vi "simulate arduino sensirion read to stream and log (sub-vi).vi"(0 "logfile refnum":refnum<file>, 1 "VISA resource name (COM3)":refnum<visa-resource-name>="COM3", 2 "stop channel":T1, 3 "abort? (F)":bool, 5 "read byte count (512)":u32=512, 7 "expected num sensors (12)":i32=12, 9 "baud rate (576000)":u32=576000, 11 "error in (no error)":errorcluster, 12 "dirty data? (F)":bool) -> (4 "logfile refnum out":refnum<file>, 8 "sensor data cluster channel":T2, 15 "error out":errorcluster)   [LabVIEW 2021]
uses:
  <extravilib>/ChannelInstances/Stream-t'sensirion_data_with_time.ctl'/)Channel.ctl
  type-defs/sensirion_data_with_time.ctl
  controls/sensirion_flow_sensor_data.ctl
  <extravilib>/ChannelInstances/Tag-bool/))Channel.ctl
  <extravilib>/ChannelInstances/Stream-t'sensirion_data_with_time.ctl'/Read With Abort.vi
  <extravilib>/ChannelInstances/Stream-t'sensirion_data_with_time.ctl'/Write With Abort.vi
  <extravilib>/ChannelInstances/Tag-bool/Read With Abort.vi
  <extravilib>/ChannelInstances/Tag-bool/Write With Abort.vi
  <extravilib>/ChannelInstances/Stream-t'sensirion_data_with_time.ctl'/EndpointRead.vi
  <extravilib>/ChannelInstances/Stream-t'sensirion_data_with_time.ctl'/Endpoint.vi
  <extravilib>/ChannelInstances/Tag-bool/EndpointRead.vi
  <extravilib>/ChannelInstances/Tag-bool/Endpoint.vi
  <extravilib>/ChannelInstances/Tag-bool/Instantiate.vi
  <extravilib>/ChannelInstances/Stream-t'sensirion_data_with_time.ctl'/Instantiate.vi
  <extravilib>/ChannelInstances/Stream-t'sensirion_data_with_time.ctl'/)Channel.vi
  <resource>/ChannelSupport/_ChannelSupport/WaitIfNeeded.vi
  <extravilib>/ChannelInstances/Stream-t'sensirion_data_with_time.ctl'.lvlib
  <extravilib>/ChannelInstances/Tag-bool.lvlib
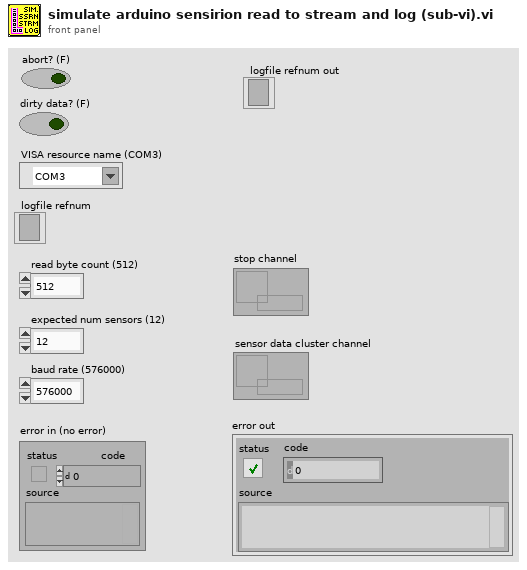
[diagram p1: front panel]
types:
  T1 = typedef "Tag-bool.lvlib/))Channel.ctl" = refnum<queue>
  T2 = typedef "Stream-t'sensirion_data_with_time.ctl'.lvlib/)Channel.ctl" = refnum<queue>
  T3 = typedef "sensirion_data_with_time.ctl" = cluster{"sensor data array":T4[], "relative timestamp":dbl, "error":errorcluster}
  T4 = typedef "sensirion_flow_sensor_data.ctl" = cluster{"flow rate \n":dbl[unit], "flow val. status":bool, "temperature":dbl[unit], "temp. val status":bool, "air in line?":bool, "high flow?":bool, "flag. val status":bool}
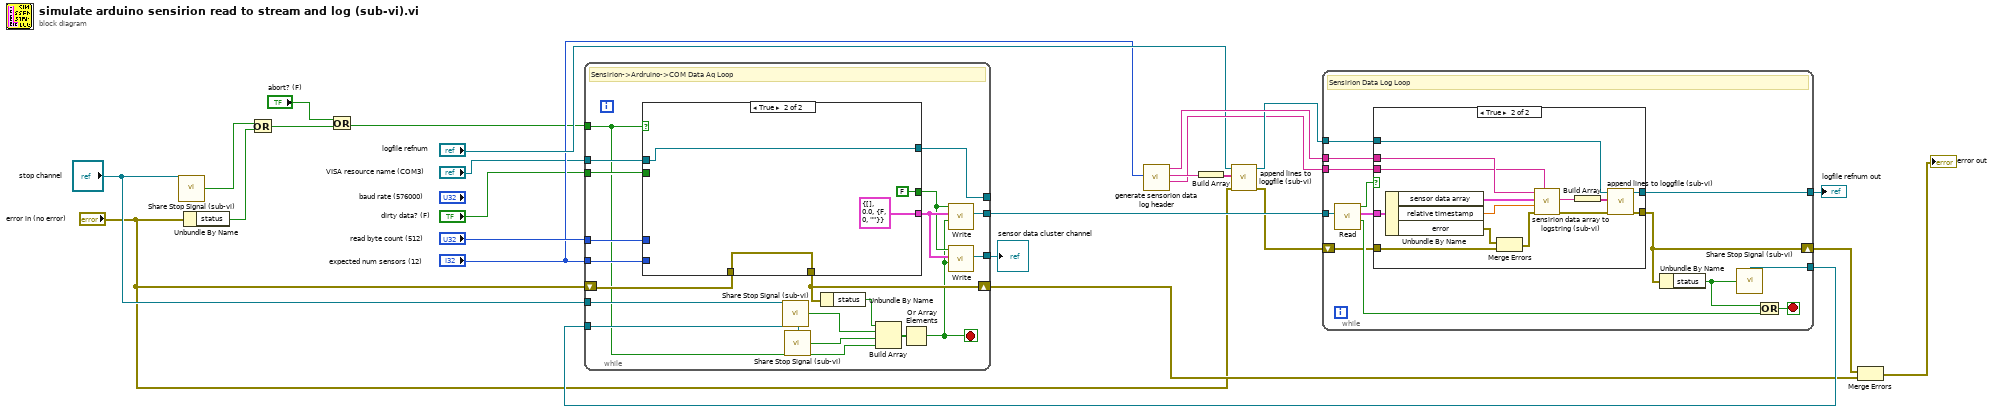
[diagram p0: block diagram]
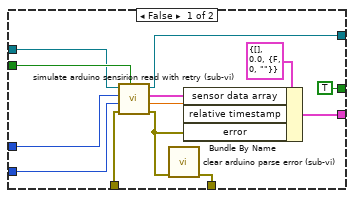
[diagram p3: hidden frame]
diagram:
  n1 = call "Share Stop Signal (sub-vi).vi"("channel"="stop channel") -> ("stop"=w8:bool)  [unwired: 1 in]
  n2 = Unbundle By Name("error in (no error)") -> ("status"=w9:bool)
  n3 = Or(x=w8, y=w9) -> (x .or. y?=w7:bool)
  n4 = Or(x="abort? (F)", y=w7) -> (x .or. y?=w4:bool)
  n5 = call "generate sensorion data log header.vi"("num sensors"="expected num sensors (12)") -> ("delimiter"=w16:string, "sensor data header string"=w25:string, "value format"=w22:string)  [unwired: 8 in]
  n6 = Build Array(w25) -> (w24:string[])
  n7 = call "append lines to loggfile (sub-vi).vi"("error in (no error)"="error in (no error)", "string array"=w24, "file refnum"="logfile refnum") -> ("error out"=w19:errorcluster, "file refnum out"=w21:refnum<file>)  [unwired: 7 in]
  n8 = while {
    tunnel: "read byte count (512)" -> [w44]
    tunnel: [w41] -> w23
    tunnel: "expected num sensors (12)" -> [w40]
    shift-right: [w37] -> w5
    shift-left: "error in (no error)" -> [w43]
    tunnel: [w39] -> w20
    tunnel: "stop channel" -> [w38]
    tunnel: [w36] -> _
    tunnel: w15 -> [w35]
    tunnel: "dirty data? (F)" -> [w34]
    tunnel: w4 -> [w28]
    tunnel: "VISA resource name (COM3)" -> [w33]
    stop <- w26 stop-if-true
    # "Sensirion->Ardruino->COM Data Aq Loop"
    n9 = case shown="True" w28 {
      tunnel: w44 -> [w57 _]
      tunnel: w43 -> [w47 w58]
      tunnel: [w53 T3 {"sensor data array"=[], "relative timestamp"=0.0, "error"={"status"=FALSE, "code"=0, "source"=""}} ("Cluster")] -> w42
      tunnel: w40 -> [w52 _]
      tunnel: [w45 w58] -> w37
      tunnel: [w51 w61] -> w36
      tunnel: w34 -> [w50 _]
      tunnel: w33 -> [w49 w61]
      tunnel: [TRUE ("element valid? (T)") FALSE ("element valid? (T)")] -> w32
      frame False {
        n10 = call "simulate arduino sensirion read with retry (sub-vi).vi"("dirty data? (F)"=w50, "error in (no error)"=w47, "expected num sensors (12)"=w52, "read byte count (512)"=w57, "VISA resource name"=w49) -> ("error out"=w46:errorcluster, "relative timestamp"=w54:dbl, "sensor data array"=w55:T4[], "VISA resource name out"=w51:refnum<visa-resource-name>)  [unwired: 2 in, 1 out]
        n11 = call "clear arduino parse error (sub-vi).vi"("error in"=w46) -> ("error out"=w45:errorcluster)  [unwired: 10 in]
        n12 = Bundle By Name(cluster=T3 {"sensor data array"=[], "relative timestamp"=0.0, "error"={"status"=FALSE, "code"=0, "source"=""}} ("Cluster"), "sensor data array"=w55, "relative timestamp"=w54, "error"=w46) -> (w53:T3)
      }
      frame True {
      }
    }
    n13 = call "Share Stop Signal (sub-vi).vi"("channel"=w38) -> ("stop"=w30:bool)  [unwired: 1 in]
    n14 = call "Share Stop Signal (sub-vi).vi"("channel"=w35) -> ("stop"=w31:bool)  [unwired: 1 in]
    n15 = Unbundle By Name(w37) -> ("status"=w29:bool)
    n16 = Build Array(w29, w30, w31, w28) -> (w27:bool[])
    n17 = Or Array Elements(Boolean array=w27) -> (logical OR=w26:bool)
    n18 = call <extravilib>:"Write.vi"("last element? (F)"=w26, "element"=w42, "element valid? (T)"=w32) -> ("channel"=w41:T2)  [unwired: 6 in, 2 out]
    n19 = call <extravilib>:"Write.vi"("last element? (F)"=w26, "element"=w42, "element valid? (T)"=w32) -> ("channel"=w39:T2)  [unwired: 6 in, 2 out]
  }
  "sensor data cluster channel" <- w20
  n20 = while {
    tunnel: w23 -> [w74]
    tunnel: w22 -> [w72]
    shift-right: [w67] -> w18
    shift-left: w19 -> [w66]
    tunnel: [w64] -> w15
    tunnel: w16 -> [w63]
    tunnel: w21 -> [w71]
    tunnel: [w70] -> w1
    stop <- w68 stop-if-true
    # "Sensirion Data Log Loop"
    n21 = call <extravilib>:"Read.vi"("channel"=w74) -> ("last element?"=w69:bool, "element"=w73:T3, "element valid?"=w62:bool)  [unwired: 6 in, 2 out]
    n22 = case shown="True" w62 {
      tunnel: w73 -> [_ w90]
      tunnel: w72 -> [_ w89]
      tunnel: w71 -> [w76 w88]
      tunnel: [w76 w83] -> w70
      tunnel: [w75 w82] -> w67
      tunnel: w66 -> [w75 w81]
      tunnel: w63 -> [_ w78]
      frame False {
      }
      frame True {
        n23 = Unbundle By Name(w90) -> ("sensor data array"=w77:T4[], "relative timestamp"=w87:dbl, "error"=w80:errorcluster)
        n24 = Merge Errors(w80, w81) -> (w79:errorcluster)
        n25 = call "sensirion data array to logstring (sub-vi).vi"("delimeter (comma)"=w78, "error in"=w79, "timestamp in relative seconds"=w87, "sensor data array"=w77, "value format (%15s)"=w89) -> ("error out"=w86:errorcluster, "string out"=w84:string)  [unwired: 5 in]
        n26 = Build Array(w84) -> (w85:string[])
        n27 = call "append lines to loggfile (sub-vi).vi"("error in (no error)"=w86, "string array"=w85, "file refnum"=w88) -> ("error out"=w82:errorcluster, "file refnum out"=w83:refnum<file>)  [unwired: 7 in]
      }
    }
    n28 = Unbundle By Name(w67) -> ("status"=w65:bool)
    n29 = call "Share Stop Signal (sub-vi).vi"("set stop (F)"=w65, "channel"=w64) -> ()  [unwired: 1 out]
    n30 = Or(x=w65, y=w69) -> (x .or. y?=w68:bool)
  }
  "logfile refnum out" <- w1
  n31 = Merge Errors(w18, w5) -> (→"error out":errorcluster)
